vi "Unit Test Parent Level Added and Removed.vi"() -> ()   [LabVIEW 2019, in "Sports Unit Tests.lvclass"]
uses:
  Sports Unit Tests.lvclass
  Classes/Michael Jordan/Michael Jordan.lvclass
  <userlib>/Blue Origin/BlueSerialization/BlueSerializer/DeserializeOptions.ctl
  <userlib>/Blue Origin/BlueSerialization/BlueSerializer/DeserializeSlicingOptions.ctl
  <userlib>/Blue Origin/BlueSerialization/BlueSerializer/DeserializeMutationOptions.ctl
  <userlib>/Blue Origin/BlueSerialization/BlueSerializer/DeserializePreservationOptions.ctl
  <userlib>/Blue Origin/BlueSerialization/BlueSerializer/PreserveNonWiredDataOption.ctl
  <vilib>/Utility/error.llb/Clear Errors.vi
  <vilib>/addons/_JKI Toolkits/Caraya/classes/Test/Define Test.vi
  <vilib>/addons/_JKI Toolkits/Caraya/classes/Assert/Assert Equal Value_Variant.vi
  <vilib>/addons/_JKI Toolkits/Caraya/classes/Assert/Assert Not Error.vi
  <vilib>/addons/_JKI Toolkits/Caraya/classes/Assert/Assert.lvclass
  <userlib>/Blue Origin/BlueSerialization/BlueSerializer/BlueSerializer.lvclass
panel:
  out "Table":string[][](table)=[["{\r  \"Class\":[\"Michael Jordan.lvclass\",\"Basketball Player.lvclass\",\"Sports Player.lvclass\",\"Human.lvclass\",\"BlueSerialization.lvlib:BlueSerializable.lvclass\"],\r  \"Version\":[\"2.0.0.3\",\"2.0.0.3\",\"2.0.0.3\",\"2.0.0.3\",\"2.0.0.0\"],\r  \"BlueSerialization.lvlib:BlueSerializable.lvclass\":{\"LibVersion\":1},\r  \"Human.lvclass\":{\r    \"alive?\":true,\r    \"Age (years)\":40,\r    \"Name\":\"M.Jordan\",\r    \"Height (ft)\":6\r  },\r  \"Sports Player.lvclass\":{\r    \"Professional?\":true,\r    \"Earnings (dollars)\":1000000,\r    \"Sponsor\":\"Nike\"\r  },\r  \"Basketball Player.lvclass\":{\r    \"Sports team\":\"Bulls\",\r    \"Free-throw percentage\":30\r  },\r  \"Michael Jordan.lvclass\":{\r    \"Latest Movie\":\"Space Jam\",\r    \"#cars owned\":6\r  }\r}", "{\r  \"Class\":[\"Michael Jordan.lvclass\",\"Golf Player.lvclass\",\"Sports Player.lvclass\",\"Human.lvclass\",\"BlueSerialization.lvlib:BlueSerializable.lvclass\"],\r  \"Version\":[\"2.0.1.6\",\"2.0.0.3\",\"2.0.0.3\",\"2.0.0.3\",\"2.0.0.0\"],\r  \"BlueSerialization.lvlib:BlueSerializable.lvclass\":{\"LibVersion\":1},\r  \"Human.lvclass\":{\r    \"alive?\":true,\r    \"Age (years)\":40,\r    \"Name\":\"Shauille O'Neal\",\r    \"Height (ft)\":6\r  },\r  \"Sports Player.lvclass\":{\r    \"Professional?\":true,\r    \"Earnings (dollars)\":1000000,\r    \"Sponsor\":\"Aladin\"\r  },\r  \"Golf Player.lvclass\":{\r    \"League\":\"\",\r    \"# holes in one\":0,\r    \"longest drive (ft)\":0\r  },\r  \"Michael Jordan.lvclass\":{\r    \"Latest Movie\":\"Space Jam\",\r    \"#cars owned\":6\r  }\r}", "Status: FALSE\ncode: 0\n", "BlueJSONTextSerializer.lvlib:BlueJSONTextSerializer.lvclass"], ["Class = [\"Michael Jordan.lvclass\", \"Basketball Player.lvclass\", \"Sports Player.lvclass\", \"Human.lvclass\", \"BlueSerialization.lvlib:BlueSerializable.lvclass\"]\r\nVersion = [\"2.0.0.3\", \"2.0.0.3\", \"2.0.0.3\", \"2.0.0.3\", \"2.0.0.0\"]\r\n\n[\"BlueSerialization.lvlib:BlueSerializable.lvclass\"]\nLibVersion = 1\r\n\n[\"Human.lvclass\"]\n\"alive?\" = true\r\n\"Age (years)\" = 40\r\nName = \"M.Jordan\"\r\n\"Height (ft)\" = 6.0\r\n\n[\"Sports Player.lvclass\"]\n\"Professional?\" = true\r\n\"Earnings (dollars)\" = 1000000.0\r\nSponsor = \"Nike\"\r\n\n[\"Basketball Player.lvclass\"]\n\"Sports team\" = \"Bulls\"\r\n\"Free-throw percentage\" = 30.0\r\n\n[\"Michael Jordan.lvclass\"]\n\"Latest Movie\" = \"Space Jam\"\r\n\"#cars owned\" = 6\r\n", "Class = [\"Michael Jordan.lvclass\", \"Golf Player.lvclass\", \"Sports Player.lvclass\", \"Human.lvclass\", \"BlueSerialization.lvlib:BlueSerializable.lvclass\"]\r\nVersion = [\"2.0.1.6\", \"2.0.0.3\", \"2.0.0.3\", \"2.0.0.3\", \"2.0.0.0\"]\r\n\n[\"BlueSerialization.lvlib:BlueSerializable.lvclass\"]\nLibVersion = 1\r\n\n[\"Human.lvclass\"]\n\"alive?\" = true\r\n\"Age (years)\" = 40\r\nName = \"Shauille O'Neal\"\r\n\"Height (ft)\" = 6.0\r\n\n[\"Sports Player.lvclass\"]\n\"Professional?\" = true\r\n\"Earnings (dollars)\" = 1000000.0\r\nSponsor = \"Aladin\"\r\n\n[\"Golf Player.lvclass\"]\nLeague = \"\"\r\n\"# holes in one\" = 0\r\n\"longest drive (ft)\" = 0.0\r\n\n[\"Michael Jordan.lvclass\"]\n\"Latest Movie\" = \"Space Jam\"\r\n\"#cars owned\" = 6\r\n", "Status: FALSE\ncode: 0\n", "BlueTOMLSerializer.lvlib:BlueTOMLSerializer.lvclass"]]
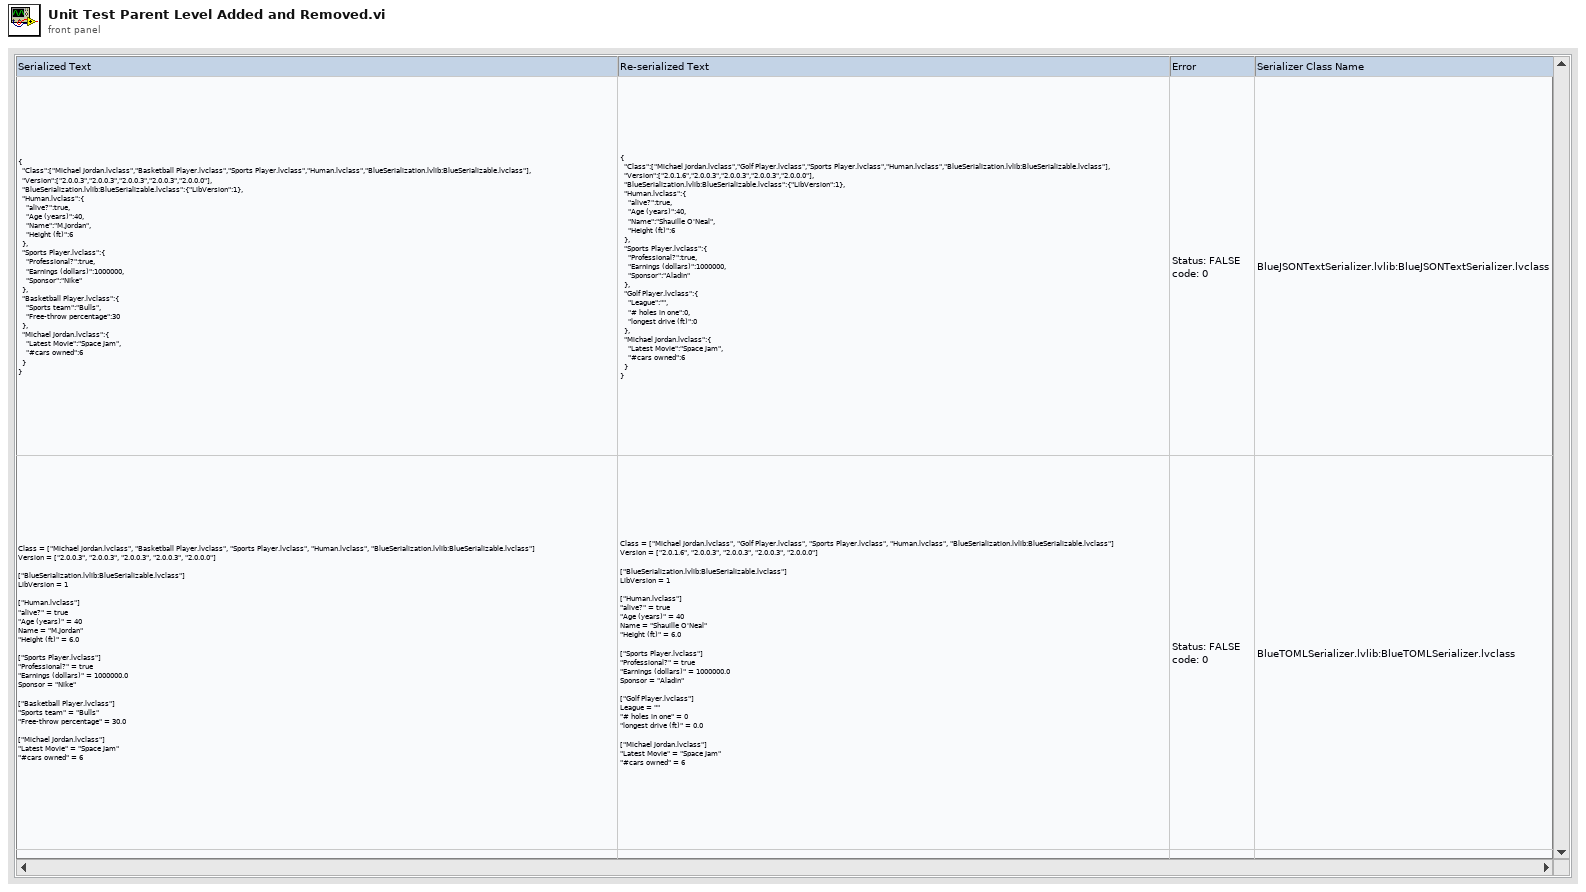
[diagram p1: front panel]
types:
  T1 = typedef "BlueSerialization.lvlib/BlueSerializer.lvclass/DeserializeOptions.ctl" = cluster{"deserialize non-BlueSerializable objects from hex?":bool, "expand objects on type conflict?":bool, "Slicing":T2, "Mutation Options":T3, "Preservation Options":T4}
  T2 = typedef "BlueSerialization.lvlib/BlueSerializer.lvclass/DeserializeSlicingOptions.ctl" = cluster{"slice flattened object data on error?":bool, "sliceable class names":string[]}
  T3 = typedef "BlueSerialization.lvlib/BlueSerializer.lvclass/DeserializeMutationOptions.ctl" = cluster{"error on inserted parent levels?":bool, "\terror on obsolete parent levels?":bool}
  T4 = typedef "BlueSerialization.lvlib/BlueSerializer.lvclass/DeserializePreservationOptions.ctl" = cluster{"Preserve wired serialized data?":bool, "Preserve wired non-serialized data":T5}
  T5 = typedef "BlueSerialization.lvlib/BlueSerializer.lvclass/PreserveNonWiredDataOption.ctl" = enum16{"Don't preserve", "Preserve (error on less-specific wired types)", "Preserve (except on less-specific wired types)"}
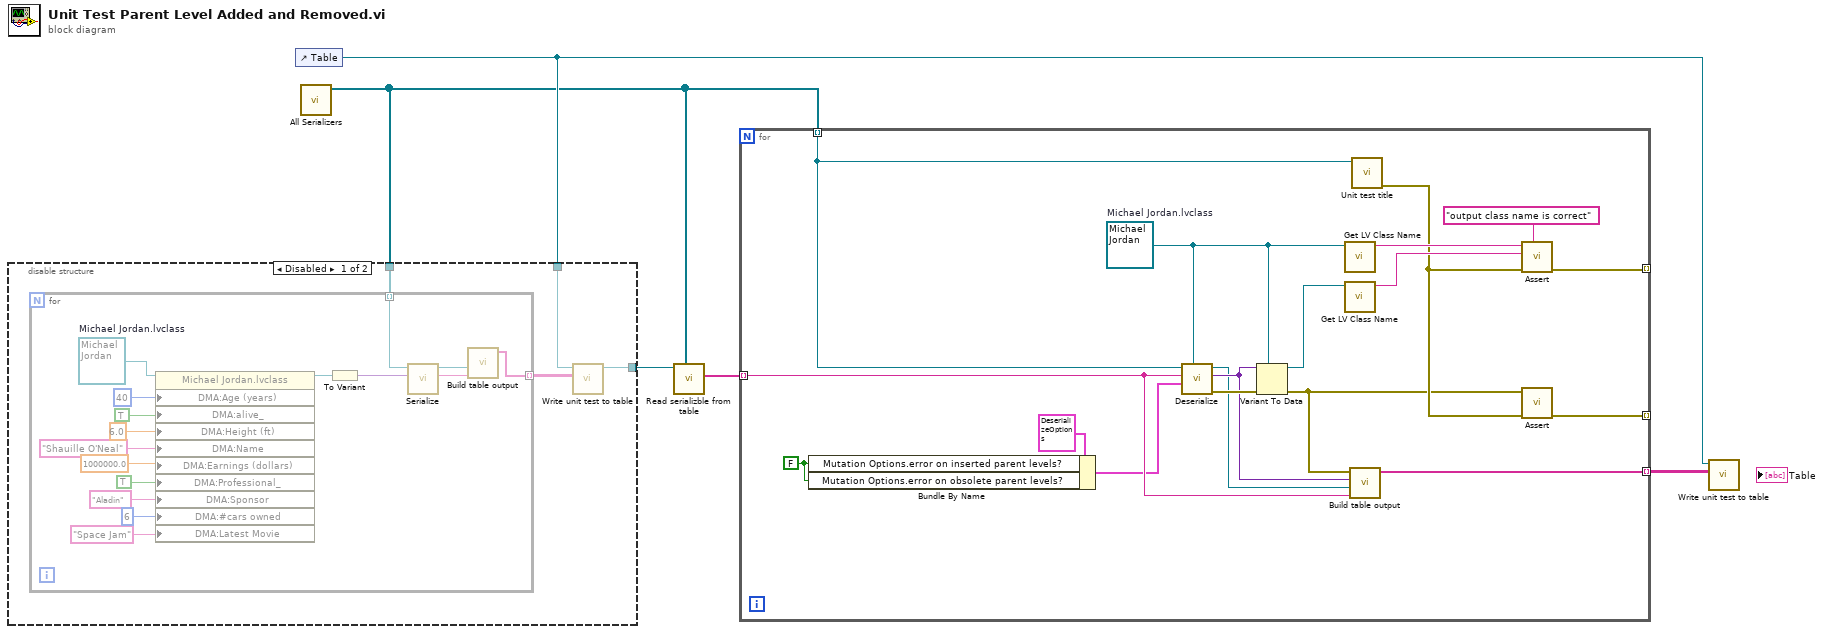
[diagram p0: block diagram]
diagram:
  n1 = control-ref of="Table"() -> (w5:refnum<vi>)
  n2 = call "All Serializers.vi"() -> ("All serializers"=w2:refnum<class "BlueSerializer.lvclass">[])  [unwired: 11 in]
  n3 = disable-structure shown="Disabled" {
    disable-tunnel: w5 -> [w8 w26]
    disable-tunnel: [w7 w26] -> w4
    disable-tunnel: w2 -> [w6 _]
    frame Disabled {
      n4 = for {
        tunnel: w6 -> [w16] mode=indexing
        tunnel: [w13] -> w9 mode=indexing
        w12 = refnum<class "Michael Jordan.lvclass"> refnum  # Michael Jordan.lvclass
        n5 = property on="Property Node" class="Michael Jordan.lvclass"(reference=w12, "DMA:Age (years)"=u16 40 ("Age (years)"), "DMA:alive_"=TRUE ("alive_"), "DMA:Height (ft)"=6.0 ("Height (ft)"), "DMA:Name"="Shauille O'Neal" ("Name"), "DMA:Earnings (dollars)"=1000000.0 ("Earnings (dollars)"), "DMA:Professional_"=TRUE ("Professional_"), "DMA:Sponsor"="Aladin" ("Sponsor"), "DMA:#cars owned"=i16 6 ("#cars owned"), "DMA:Latest Movie"="Space Jam" ("Latest Movie")) -> (reference out=w25:refnum<class "Michael Jordan.lvclass">)  [unwired: 1 in, 1 out]
        n6 = To Variant(anything=w25) -> (Variant=w17:variant)
        n7 = call <userlib>:"Serialize.vi"("Anything"=w17, "BlueSerializer in"=w16) -> ("Serialized Text"=w15:string, "BlueSerializer out"=w14:refnum<class "BlueSerializer.lvclass">)  [unwired: 7 in, 1 out]
        n8 = call "Build table output.vi"("serialized text"=w15, "BlueSerializer in"=w14) -> ("table output"=w13:string[])  [unwired: 9 in]
      }
      n9 = call "Write unit test to table.vi"("Table"=w9, "Table ref in"=w8) -> ("Table ref out"=w7:refnum<vi>)  [unwired: 9 in]
    }
    frame Enabled {
    }
  }
  n10 = call "Read serializble from table.vi"("serializers"=w2, "Table ref in"=w4) -> ("serializable texts"=w3:string[])  [unwired: 7 in, 2 out]
  n11 = for {
    tunnel: w2 -> [w28] mode=indexing
    tunnel: [w39] -> _ mode=indexing
    tunnel: [w38] -> _ mode=indexing
    tunnel: w3 -> [w33] mode=indexing
    tunnel: [w32] -> w1 mode=indexing
    w29 = FALSE ("Allow class expansion?")
    w31 = refnum<class "Michael Jordan.lvclass"> refnum  # Michael Jordan.lvclass
    n12 = Bundle By Name(cluster=T1 {"deserialize non-BlueSerializable objects from hex?"=FALSE, "expand objects on type conflict?"=FALSE, "Slicing"={"slice flattened object data on error?"=FALSE, "sliceable class names"=[]}, "Mutation Options"={"error on inserted parent levels?"=FALSE, "\terror on obsolete parent levels?"=FALSE}, "Preservation Options"={"Preserve wired serialized data?"=FALSE, "Preserve wired non-serialized data"=enum."Don't preserve"}} ("Deserialize Options"), "Mutation Options.error on inserted parent levels?"=w29, "Mutation Options.error on obsolete parent levels?"=w29) -> (w27:T1)
    n13 = call <userlib>:"Deserialize.vi"("Anything"=w31, "Deserialize Options"=w27, "Serialized Text"=w33, "BlueSerializer in"=w28) -> ("error out"=w44:errorcluster, "Variant"=w35:variant, "BlueSerializer out"=w34:refnum<class "BlueSerializer.lvclass">)  [unwired: 5 in]
    n14 = Variant To Data(error in=w44, type=w31, Variant=w35) -> (data=w43:refnum<class "Michael Jordan.lvclass">, error out=w36:errorcluster)
    n15 = call <vilib>:"Get LV Class Name.vi"("object"=w31) -> ("class name"=w42:string)  [unwired: 9 in, 1 out]
    n16 = call <vilib>:"Get LV Class Name.vi"("object"=w43) -> ("class name"=w41:string)  [unwired: 9 in, 1 out]
    n17 = call "Build table output.vi"("serialized text"=w33, "BlueSerializer in"=w34, "deserialized variant"=w35, "variant to data error"=w36) -> ("table output"=w32:string[])  [unwired: 7 in]
    n18 = call "Unit test title.vi"("serializer"=w28) -> ("error out"=w37:errorcluster)  [unwired: 9 in, 1 out]
    n19 = call-poly <vilib>:"Assert.vi"("Label"="output class name is correct", "error in (no error)"=w37, "Y"=w41, "X"=w42) -> ("error out"=w38:errorcluster)  [unwired: 7 in]
    n20 = call-poly <vilib>:"Assert.vi"("error in (no error)"=w37, "Not Error?"=w36) -> ("error out"=w39:errorcluster)  [unwired: 9 in]
  }
  n21 = call "Write unit test to table.vi"("Table"=w1, "Table ref in"=w5) -> ()  [unwired: 9 in, 1 out]
